vi "Logic_Config_Device.vi"(4 "error in (no error)":errorcluster, 5 "Analog Config":T1={"Enable Analog Channels"=[], "Analog Sample Rate (Samp/Sec)"=6250000} {"Analog Sample Rate (Samp/Sec)" format="%#.4p"}, 6 "Digital Config":T2={"Enable Digital Channels"=[], "Digital Sample Rate (Samp/Sec)"=10000000, "Digital Threshold(V)"=3.3000000000000007} {"Digital Threshold(V)" format="%#_13g"; "Digital Sample Rate (Samp/Sec)" format="%.0p"}, 7 "Session Ref In":T3) -> (0 "error out":errorcluster, 3 "Session Ref Out":T3)   [LabVIEW 2021]
panel:
  # "Options: 50M, 12.5M, 6.25M, 3.125M, 1.5625M, 781.25k, 31.25k, 15.625k, 6.25k, 1.25k, 250, 50\n(Analog and Digital Rates must be multiples)"
  # "Options: 500M, 250M, 125M, 100M, 10M 6.25M S/s\n(Analog and Digital Rates must be multiples)"
  # "Options: 3.3, 1.8, 1.2 V"
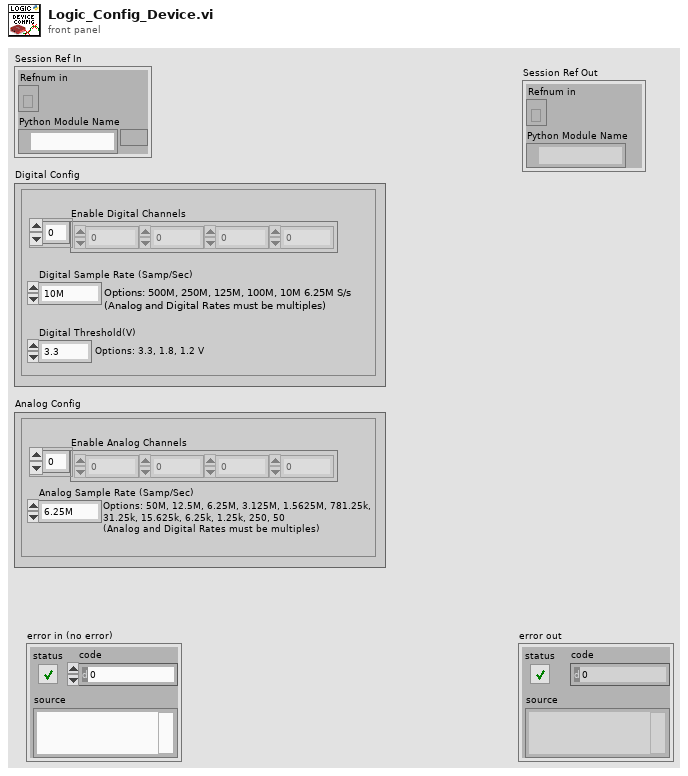
[diagram p1: front panel]
types:
  T1 = cluster{"Enable Analog Channels":i32[], "Analog Sample Rate (Samp/Sec)":i32}
  T2 = cluster{"Enable Digital Channels":i32[], "Digital Sample Rate (Samp/Sec)":i32, "Digital Threshold(V)":dbl}
  T3 = cluster{"Refnum in":refnum<k35>, "Python Module Name":path}
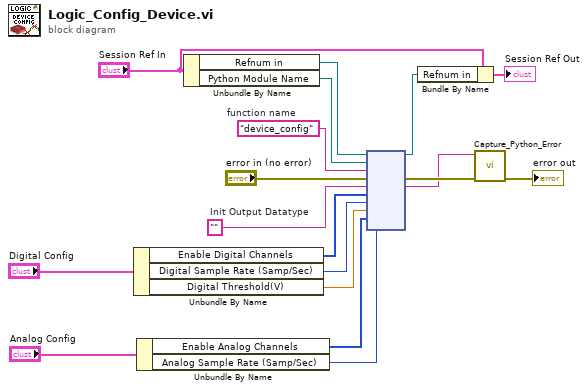
[diagram p0: block diagram]
diagram:
  w17 = "device_config"  # function name
  w16 = ""  # Init Output Datatype
  n1 = Unbundle By Name("Digital Config") -> ("Enable Digital Channels"=w9:i32[], "Digital Sample Rate (Samp/Sec)"=w7:i32, "Digital Threshold(V)"=w8:dbl)
  n2 = Unbundle By Name("Analog Config") -> ("Enable Analog Channels"=w5:i32[], "Analog Sample Rate (Samp/Sec)"=w4:i32)
  n3 = Unbundle By Name("Session Ref In") -> ("Refnum in"=w15:refnum<k35>, "Python Module Name"=w14:path)
  n4 = node(w15, w14, w17, "error in (no error)", w16, w9, w7, w8, w5, w4) -> (w12:refnum<k35>, w2:errorcluster, w1:string)  [unwired: 5 in, 2 out]
  n5 = Bundle By Name(cluster="Session Ref In", "Refnum in"=w12) -> (→"Session Ref Out":T3)
  n6 = call "Capture_Python_Error.vi"("error in (no error)"=w2, "Error Message (start with ERROR)"=w1) -> ("error out"=→"error out":errorcluster)  [unwired: 9 in]
